vi "Available Maze Levels.vi"(11 "MazeGen Folder":path) -> (3 "Available Maze Levels":string[](array[string]))   [LabVIEW 2020, in "Maze.lvlib" / "MazeGen.lvclass"]
uses:
  MazeGen.lvclass
  <vilib>/Utility/LVLibp/NI_PackedLibraryUtility.lvlib
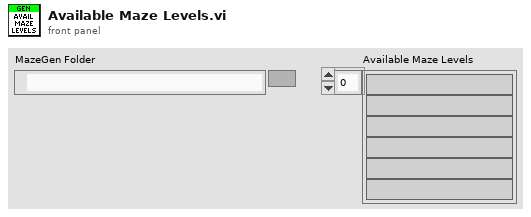
[diagram p1: front panel]
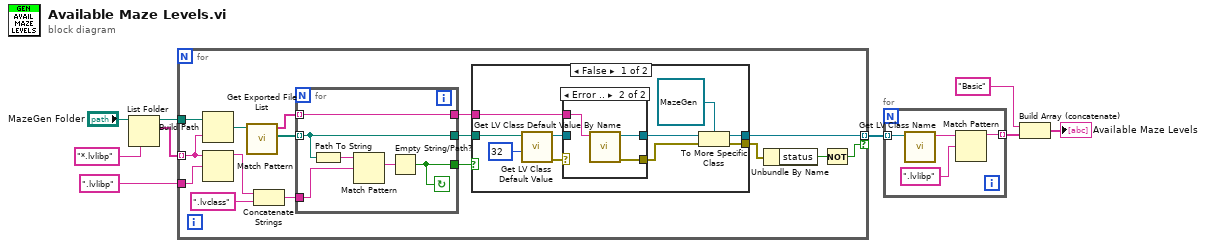
[diagram p0: block diagram]
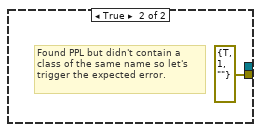
[diagram p3: hidden frame]
diagram:
  n1 = List Folder(path="MazeGen Folder", pattern="*.lvlibp") -> (path out=w8:path, filenames=w7:string[])  [unwired: 2 in, 2 out]
  n2 = for {
    tunnel: w8 -> [w20]
    tunnel: w7 -> [w12] mode=indexing
    tunnel: [w16] -> w6 mode=indexing if=w13
    tunnel: ".lvlibp" ("pattern") -> [w11]
    n3 = Build Path(base path=w20, name or relative path=w12) -> (appended path=w19:path)
    n4 = Match Pattern(string=w12, regular expression=w11) -> (before substring=w10:string)  [unwired: 1 in, 3 out]
    n5 = call <vilib>:"Get Exported File List.vi"("packed library path"=w19) -> ("paths"=w25:path[], "qualified names"=w22:string[])  [unwired: 8 in, 1 out]
    n6 = Concatenate Strings(w10, ".lvclass" ("string")) -> (w17:string)
    n7 = for {
      tunnel: w25 -> [w46] mode=indexing
      tunnel: [w46] -> w23
      tunnel: w17 -> [w44]
      tunnel: [w42] -> w24
      tunnel: w22 -> [w41] mode=indexing
      tunnel: [w41] -> w21
      stop <- w42 continue-if-true
      n8 = Path To String(path=w46) -> (string=w45:string)
      n9 = Match Pattern(string=w45, regular expression=w44) -> (match substring=w43:string)  [unwired: 1 in, 3 out]
      n10 = Empty String/Path?(string/path=w43) -> (empty?=w42:bool)
    }
    n11 = case shown="False" w24 {
      tunnel: w23 -> [w35 _]
      tunnel: w21 -> [w32 _]
      tunnel: [w28 _] -> w16
      tunnel: [w26 errorcluster {"status"=TRUE, "code"=1, "source"=""} ("error out")] -> w15
      frame False {
        n12 = call <vilib>:"Get LV Class Default Value.vi"("options"=u32 32, "class path"=w35) -> ("error out"=w33:errorcluster, "object"=w31:refnum<class>)  [unwired: 8 in]
        n13 = case shown="Error .." w33 {
          tunnel: w32 -> [_ w39]
          tunnel: w31 -> [w36 _]
          tunnel: [w36 w38] -> w30
          tunnel: [_ w37] -> w27
          frame No Error {
          }
          frame Error {
            n14 = call <vilib>:"Get LV Class Default Value By Name.vi"("class name"=w39) -> ("error out"=w37:errorcluster, "object"=w38:refnum<class>)  [unwired: 9 in]
          }
        }
        n15 = To More Specific Class(target class=refnum<class "MazeGen.lvclass"> refnum ("Maze.lvlib:MazeGen.lvclass"), reference=w30, error in=w27) -> (specific class reference=w28:refnum<class "MazeGen.lvclass">, error out=w26:errorcluster)
      }
      frame True {
        # "Found PPL but didn't contain a class of the same name so let's trigger the expected error."
      }
    }
    n16 = Unbundle By Name(w15) -> ("status"=w14:bool)
    n17 = Not(x=w14) -> (.not. x?=w13:bool)
  }
  n18 = for {
    tunnel: w6 -> [w50] mode=indexing
    tunnel: [w47] -> w5 mode=indexing
    n19 = call <vilib>:"Get LV Class Name.vi"("object"=w50) -> ("class name"=w49:string)  [unwired: 9 in, 1 out]
    n20 = Match Pattern(string=w49, regular expression=".lvlibp") -> (before substring=w47:string)  [unwired: 1 in, 3 out]
  }
  n21 = Build Array (concatenate)("Basic", w5) -> (→"Available Maze Levels":string[])
